vi "Multiprocessing_VI.vi"() -> ()   [LabVIEW 2022 SP3]
uses:
  <vilib>/Analysis/baseanly.llb/Mean (DBL).vi
  <vilib>/DAQmx/read.llb/DAQmx Read (Analog 1D Wfm NChan NSamp).vi
  <vilib>/addons/control/pid/pid.llb/PID Gain Schedule (DBL).vi
  STOP_GLOBAL.vi
  <vilib>/DAQmx/configure/timing.llb/DAQmx Timing (Sample Clock).vi
  <vilib>/DAQmx/miscellaneous.llb/DAQmx Fill In Error Info.vi
  <resource>/objmgr/daqmx.rc
  <vilib>/addons/control/pid/NI_PID_pid.lvlib
  <vilib>/Analysis/NI_AALBase.lvlib
panel:
  in  "Filename":path=path "C:/1. Rocket Research Project/CollectedData/Plots/TestingData.lvm"
  out "Vol Flow":cluster{dbl[], dbl[]}(graph)
  out "Chamber Pressure":cluster{dbl[], dbl[]}(graph)
  out "Inlet Pressure":cluster{dbl[], dbl[]}(graph)
  out "Line Pressure":cluster{dbl[], dbl[]}(graph)
  out "Waveform Chart":cluster{"mean":dbl, "MV":dbl}(graph)
  out "number of samples written per channel":u32
  in  "stop 2":bool
  in  "stop":bool
  out "Voltage Out Array":dbl[](array[numeric])
  out "SampClk.Rate 2":dbl
  out "Output":dbl(slide)=30.8641975308642 scale=0.0..5.067 scale format="%.1f"
  in  "Automatic":bool=TRUE
  in  "SP":dbl
  in  "MV":dbl(slide)=30.8641975308642 scale=0.0..5.067 scale format="%.1f"
  in  "PID gain schedule":T1(array[cluster])=[{"PID gains"={"proportional gain (Kc)"=1.0, "integral time (Ti, min)"=0.01, "derivative time (Td, min)"=0.0}, "max value"=100.0}] {"max value" format="%.2f"; "PID gains"."derivative time (Td, min)" format="%.3f"; "PID gains"."integral time (Ti, min)" format="%.3f"; "PID gains"."proportional gain (Kc)" format="%.3f"}
  out "Supply Pressure":dynamicdata(graph)
  out "Inlet Pressure":dynamicdata(graph)
  out "Line Pressure":dynamicdata(graph)
  out "Chamber Pressure PSI":dynamicdata(graph)
  out "Waiting \nfor Start":bool=TRUE
  in  "Start VI":bool
  out "SampClk.Rate":dbl
  in  "Sample Number":i32=100
  in  "Channel Control":bool[](array[boolean])
  in  "Rate":dbl=1000.0 format="%0.2f"
  out "Time":dbl
  out "Supply Pressure":cluster{dbl[], dbl[]}(graph)
  out "x*y":i32
  out "error out":errorcluster
  out "Iterations":i32
  in  "Collect?":bool=TRUE caption="Enable"
  out "Thrust 3":dynamicdata(graph)
  out "Thrust 2":dynamicdata(graph)
  out "Vertical Stand Thrust":dynamicdata(graph)
  out "AI7":dynamicdata(graph)
  out "AI6":dynamicdata(graph)
  out "AI5":dynamicdata(graph)
  out "Voltage Output":dynamicdata(graph)
  out "Temperature":dynamicdata(graph)
  out "Vol Flow L/min":dynamicdata(graph)
  in  "main":bool
  # "Pressure Channels"
  # "DAQ Configuration"
  # "AI 0 - Supply Pressure"
  # "AI 1 - Line Pressure"
  # "AI 2 - Inlet Pressure"
  # "AI 3 - Chamber Pressure"
  # "AI 4 - Volumetric Flow"
  # "AI 5"
  # "AI 6"
  # "AI 7 - Voltage"
  # "Thrust 1"
  # "Thrust 2"
  # "Thrust 3"
  # "Temperature"
  # "Thrust Channels"
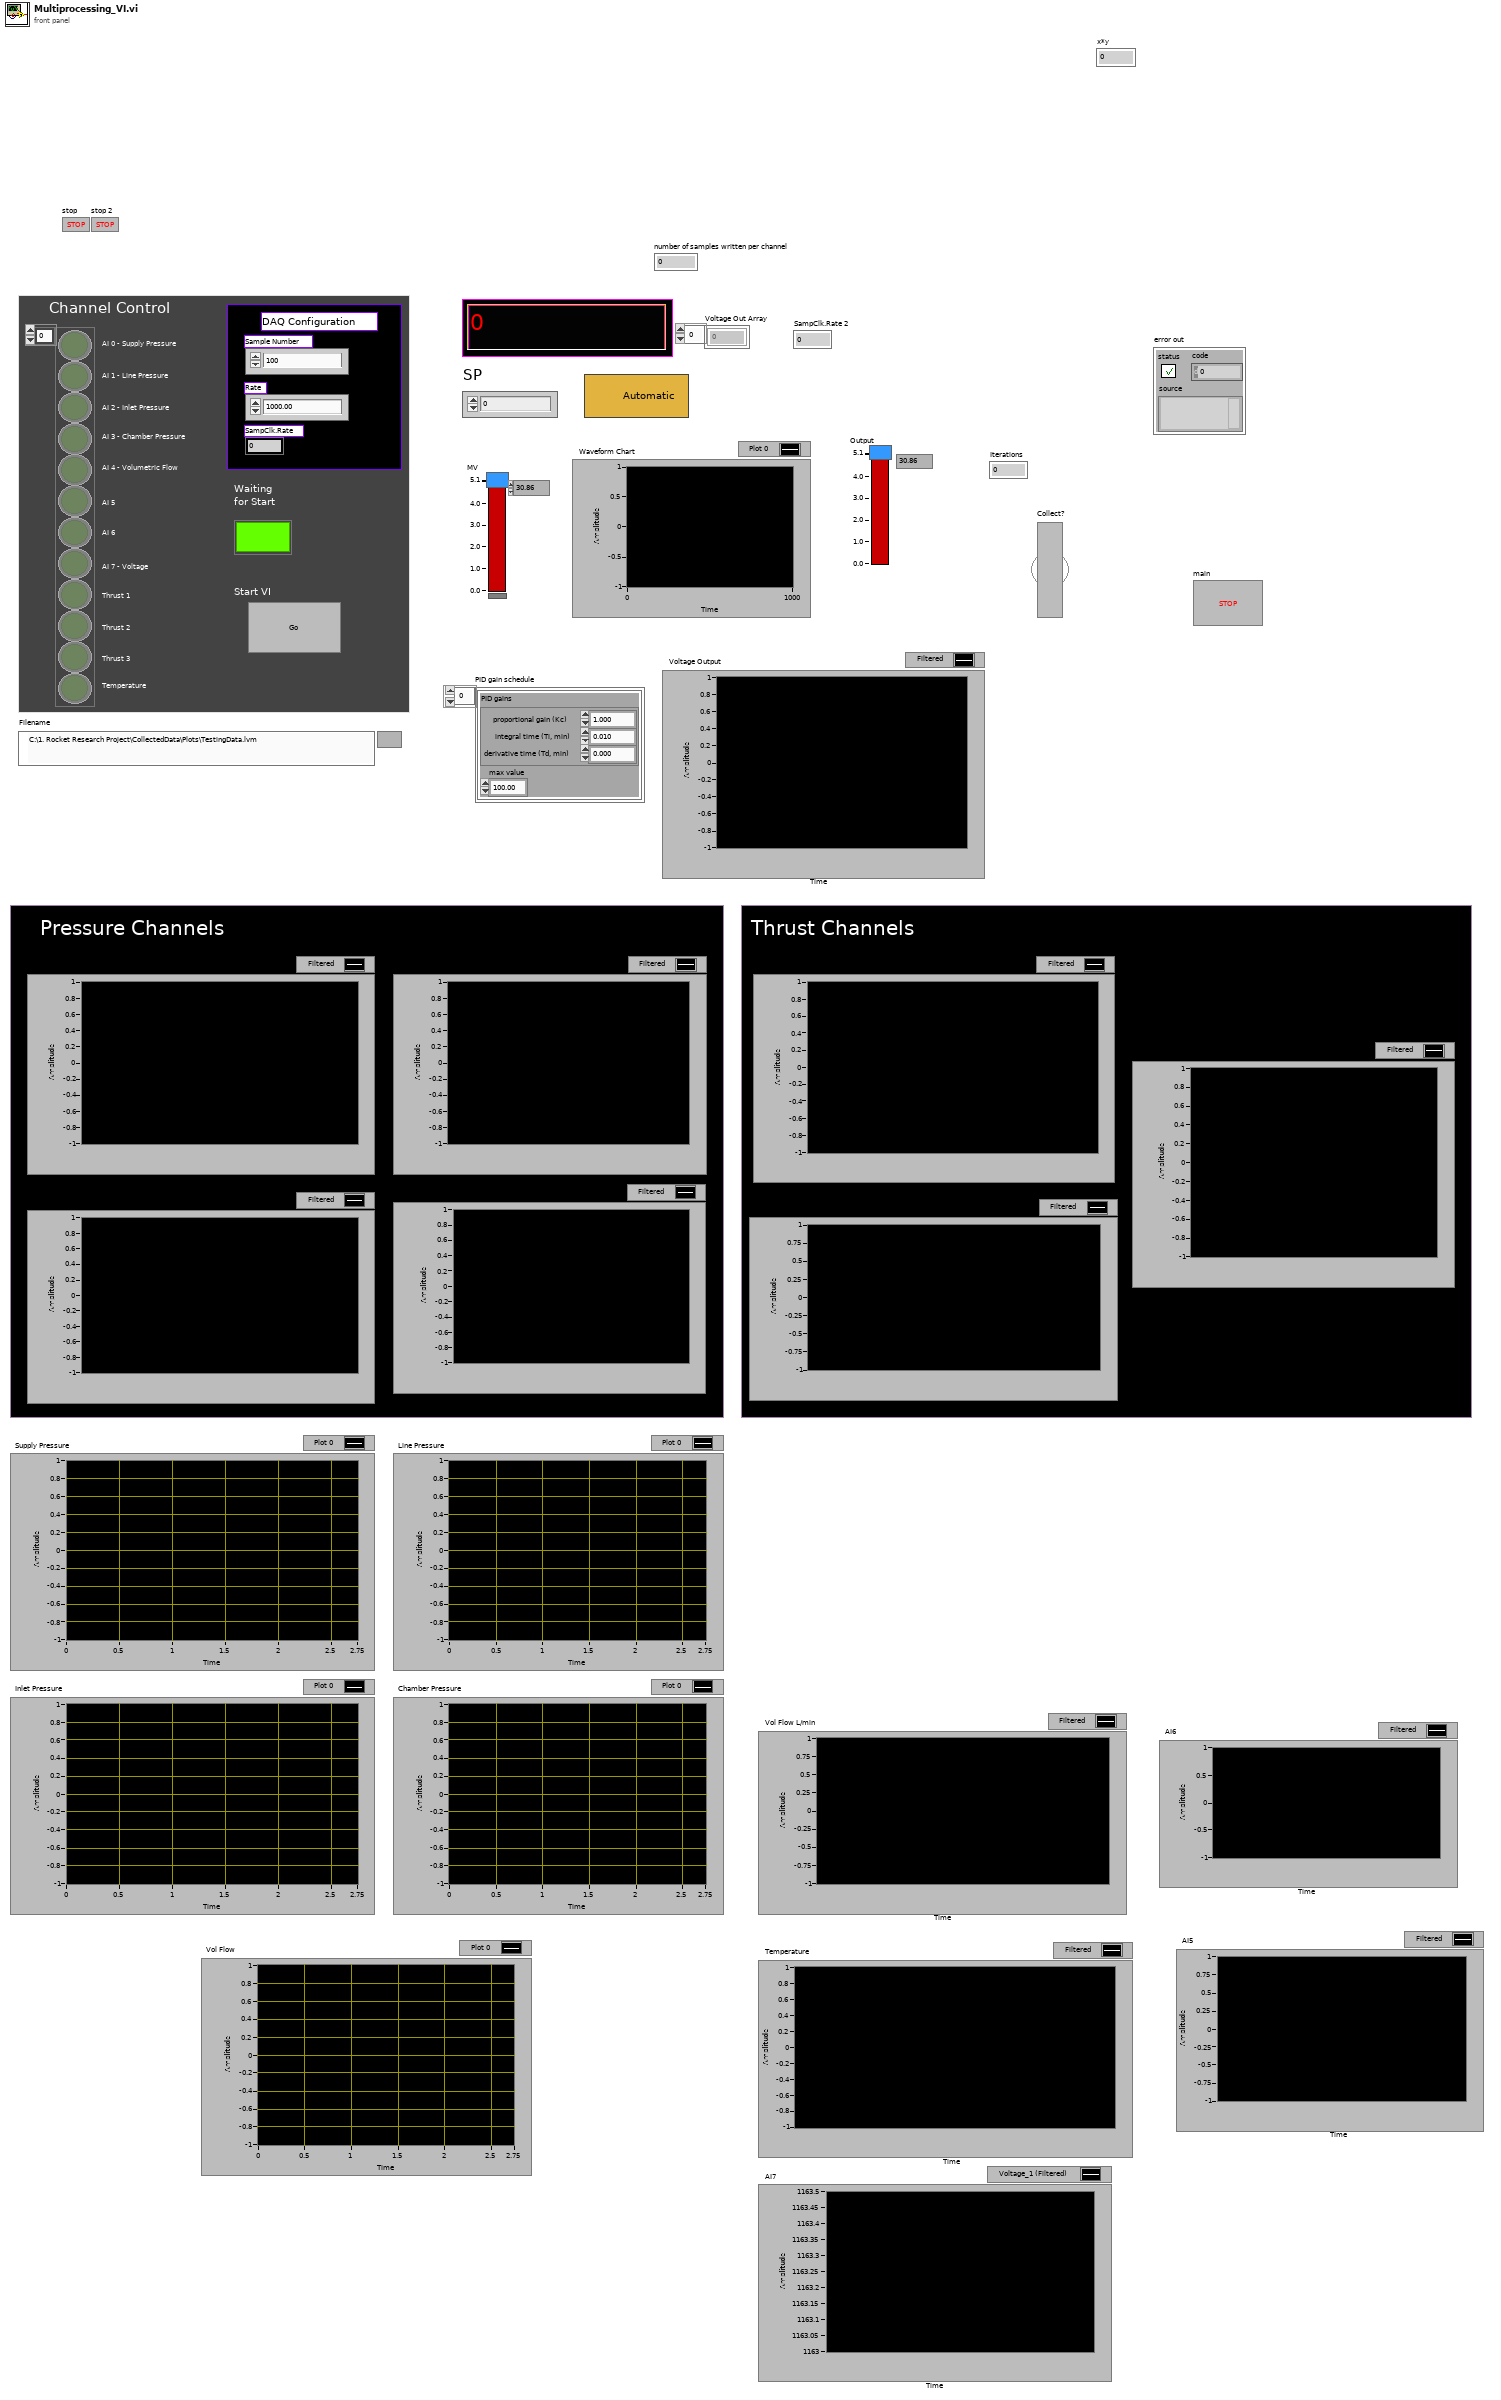
[diagram p1: front panel]
types:
  T1 = cluster{"PID gains":cluster{"proportional gain (Kc)":dbl, "integral time (Ti, min)":dbl, "derivative time (Td, min)":dbl}, "max value":dbl}[]
  T2 = cluster{"Modulus":dbl, "Number of\nComplete Cycles":dbl}
  T3 = cluster{"Dynamic Data":dynamicdata, "Dynamic Data":dynamicdata, "Dynamic Data":dynamicdata, "Dynamic Data":dynamicdata, "Dynamic Data":dynamicdata, "Dynamic Data":dynamicdata, "Dynamic Data":dynamicdata, "Dynamic Data":dynamicdata, "Dynamic Data":dynamicdata, "Dynamic Data":dynamicdata, "Dynamic Data":dynamicdata, "Dynamic Data":dynamicdata}
  T4 = cluster{"PID gains":cluster{"Kc":dbl, "Ti":dbl, "Td":dbl}, "max value":dbl}[]
  T5 = cluster{"proportional gain (Kc)":dbl, "integral time (Ti, min)":dbl, "derivative time (Td, min)":dbl}
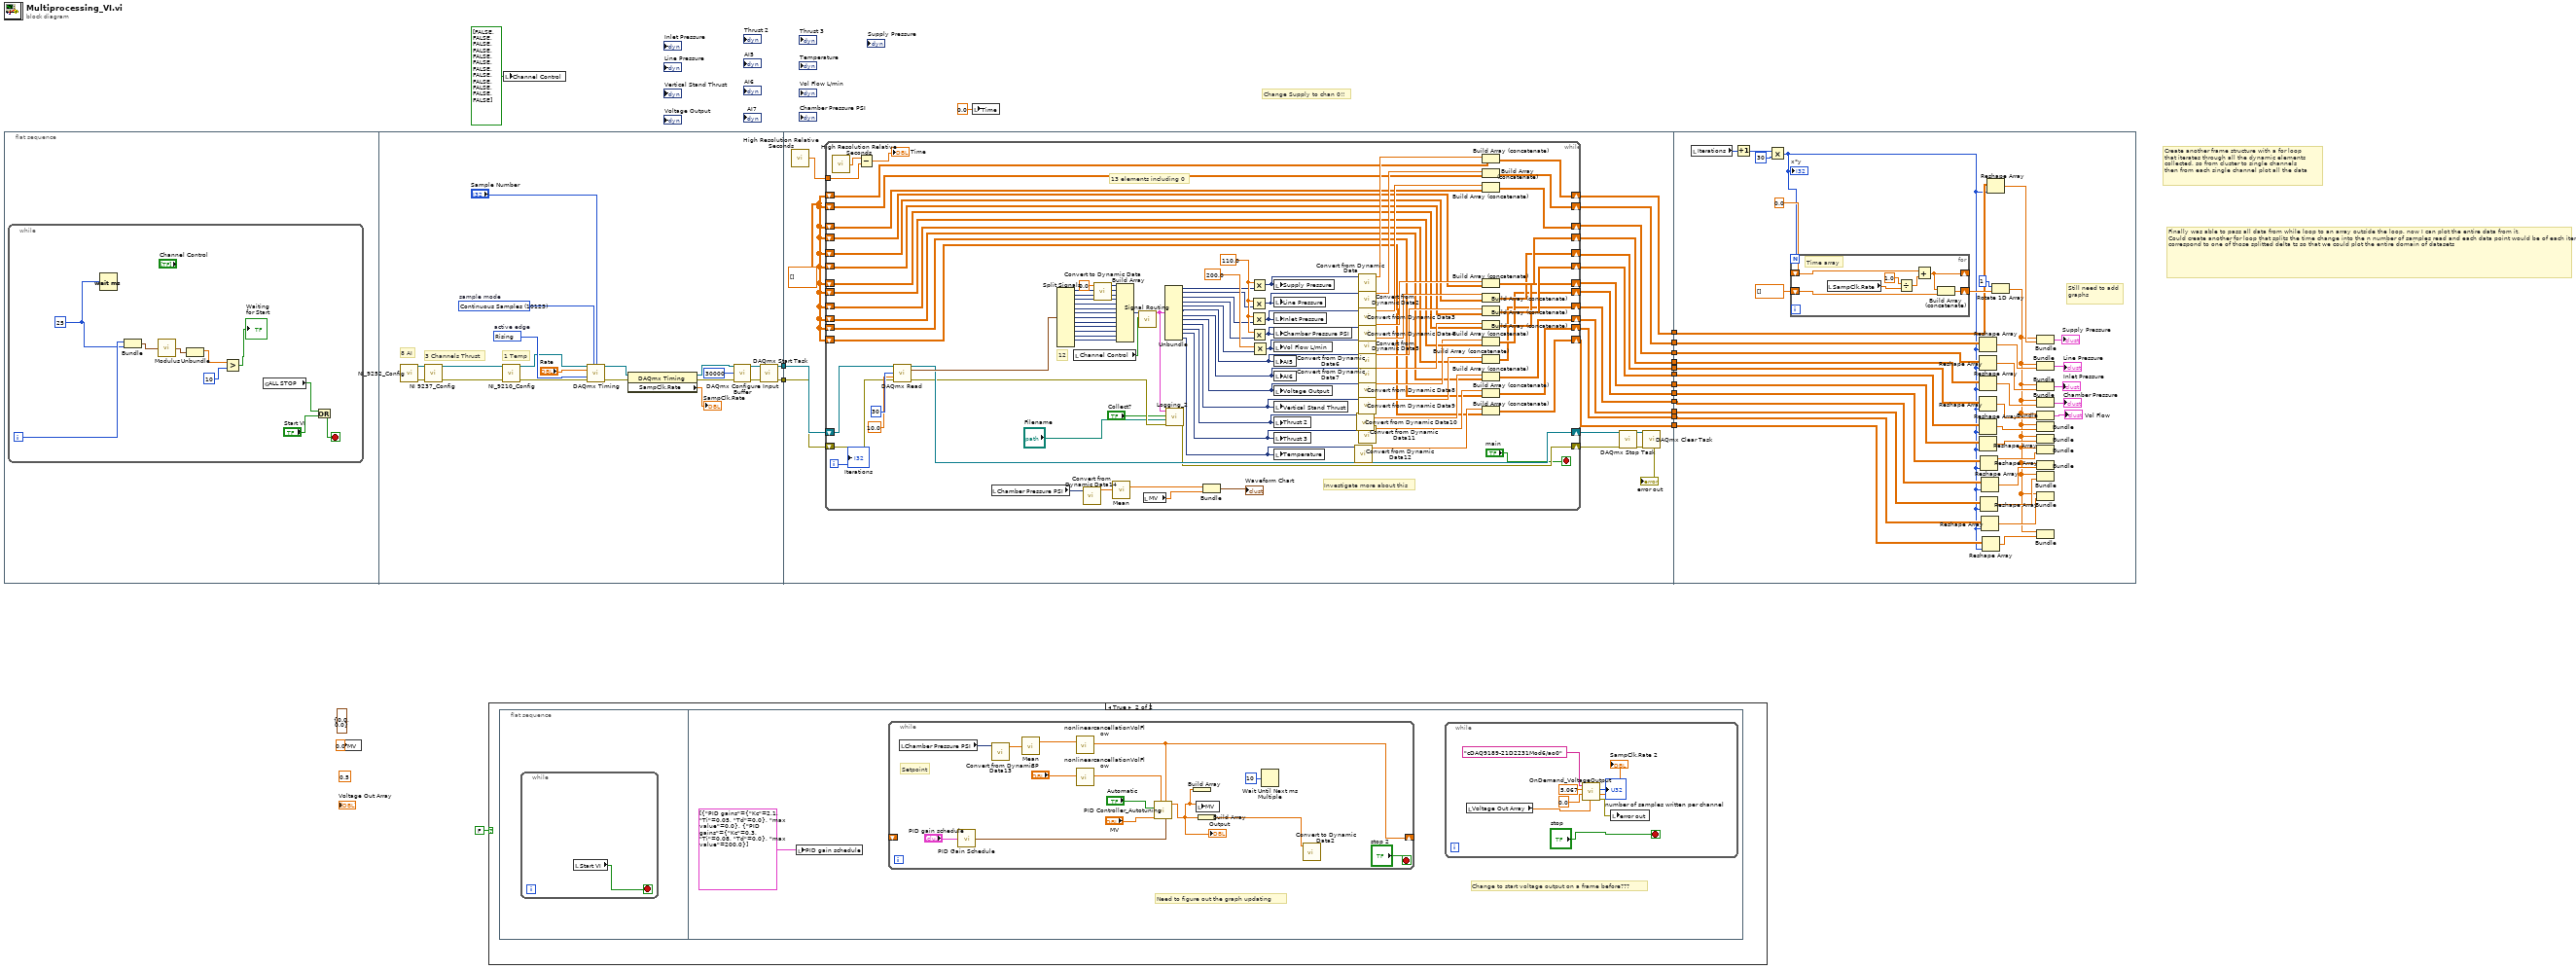
[diagram p0: block diagram]
diagram:
  (unwired) cluster{"initial PV":dbl, "setpoint":dbl} {"initial PV"=0.0, "setpoint"=0.0} ("PV Setpoint Output")
  (unwired) 0.5 ("X Scale.Offset and Multiplier:Multiplier")
  # "Change Supply to chan 0!!"
  # "Finally was able to pass all data from while loop to an array outside the loop, now I can plot the entire data from it, \nCould create another for loop that splits the time change into the n number of samples read and each data point would be of each iteration would correspond to one of those splitted delta ts so that we could plot the entire domain of datasets"
  # "Create another frame structure with a for loop\nthat iterates through all the dynamic elements\ncollected, so from cluster to single channels\nthen from each single channel plot all the data"
  n1 = flat-sequence {
    tunnel: [w34] -> w17
    tunnel: [w33] -> w16
    tunnel: w17 -> [w69]
    tunnel: w16 -> [w68]
    tunnel: [w61] -> w15
    tunnel: [w59] -> w13
    tunnel: [w58] -> w12
    tunnel: [w57] -> w11
    tunnel: [w56] -> w10
    tunnel: [w55] -> w9
    tunnel: [w54] -> w8
    tunnel: [w53] -> w7
    tunnel: [w52] -> w6
    tunnel: [w51] -> w5
    tunnel: [w50] -> w4
    tunnel: [w49] -> w3
    tunnel: w15 -> [w190]
    tunnel: w13 -> [w189]
    tunnel: w12 -> [w188]
    tunnel: w11 -> [w187]
    tunnel: w10 -> [w186]
    tunnel: w9 -> [w185]
    tunnel: w8 -> [w184]
    tunnel: w7 -> [w177]
    tunnel: w6 -> [w175]
    tunnel: w5 -> [w173]
    tunnel: w4 -> [w171]
    tunnel: w3 -> [w167]
    frame #0 {
      n2 = while {
        i -> [w28]
        stop <- w20 stop-if-true
        w19 = u32 25 ("milliseconds to wait")
        n3 = Wait (ms)(milliseconds to wait=w19) -> ()  [unwired: 1 out]
        n4 = Bundle(w28, "milliseconds to wait"=w19) -> (w27:cluster{i32, "milliseconds to wait":u32})  [unwired: 1 in]
        n5 = call "Modulus.vi"("Input"=w27) -> ("Output"=w26:T2)
        n6 = Unbundle(w26) -> ("Modulus"=w25:dbl)  [unwired: 1 out]
        n7 = Greater?(x=w25, y=u32 10 ("milliseconds to wait")) -> (0:→"Waiting \nfor Start":bool)
        n8 = global read "STOP_GLOBAL.vi" "ALL STOP"() -> (w22:bool)
        n9 = Or(x=w22, y="Start VI") -> (x .or. y?=w20:bool)
      }
    }
    frame #1 {
      w38 = 10123 items=["Finite Samples"=10178, "Continuous Samples"=10123, "Hardware Timed Single Point"=12522]  # sample mode
      w37 = 10280 items=["Rising"=10280, "Falling"=10171]  # active edge
      # "1 Temp"
      # "8 AI"
      # "3 Channels Thrust"
      n10 = call "NI_9252_Config.vi"() -> ("error out"=w31:errorcluster, "task out"=w32:refnum<k21>)  [unwired: 10 in]
      n11 = call "NI 9237_Config.vi"("error in"=w31, "task in"=w32) -> ("error out"=w48:errorcluster, "task out"=w47:refnum<k21>)  [unwired: 8 in]
      n12 = call "NI_9210_Config.vi"("error in"=w48, "task in"=w47) -> ("error out"=w30:errorcluster, "task out"=w29:refnum<k21>)  [unwired: 8 in]
      n13 = call-poly <vilib>:"DAQmx Timing.vi"("task/channels in"=w29, "sample mode"=w38, "samples per channel"="Sample Number", "rate"="Rate", "active edge"=w37, "error in"=w30) -> ("task out"=w41:refnum<k21>, "error out"=w42:errorcluster)  [unwired: 8 in]
      n14 = property class="DAQmx Timing"(reference=w41, error in=w42) -> (reference out=w43:refnum<k21>, error out=w44:errorcluster, "SampClk.Rate"=→"SampClk.Rate":dbl)
      n15 = call <vilib>:"DAQmx Configure Input Buffer.vi"("task/channels in"=w43, "buffer size (in samples per channel)"=u32 30000, "error in"=w44) -> ("task out"=w46:refnum<k21>, "error out"=w45:errorcluster)  [unwired: 11 in]
      n16 = call <vilib>:"DAQmx Start Task.vi"("task/channels in"=w46, "error in"=w45) -> ("task out"=w34:refnum<k21>, "error out"=w33:errorcluster)  [unwired: 12 in]
    }
    frame #2 {
      w60 = dbl[][] []
      n17 = call <vilib>:"High Resolution Relative Seconds.vi"() -> ("relative seconds"=w67:dbl)
      n18 = while {
        shift-right: [w156] -> w63
        shift-left: w69 -> [w158]
        shift-right: [w131] -> w62
        shift-left: w68 -> [w157]
        shift-right: [w123] -> w61
        shift-left: w60 -> [w76]
        tunnel: w67 -> [w126]
        shift-right: [w117] -> w59
        shift-left: w60 -> [w118]
        shift-right: [w111] -> w58
        shift-left: w60 -> [w112]
        shift-right: [w109] -> w57
        shift-left: w60 -> [w110]
        shift-right: [w106] -> w56
        shift-left: w60 -> [w105]
        shift-right: [w99] -> w55
        shift-left: w60 -> [w97]
        shift-right: [w98] -> w54
        shift-left: w60 -> [w96]
        shift-right: [w95] -> w53
        shift-left: w60 -> [w94]
        shift-right: [w88] -> w52
        shift-left: w60 -> [w87]
        shift-right: [w86] -> w51
        shift-left: w60 -> [w85]
        shift-right: [w82] -> w50
        shift-left: w60 -> [w81]
        shift-right: [w78] -> w49
        shift-left: w60 -> [w77]
        i -> [w129]
        stop <- "main" stop-if-true
        w139 = 110.0 ("x")
        # "Investigate more about this"
        # "13 elements including 0"
        # "12"
        n19 = call <vilib>:"High Resolution Relative Seconds.vi"() -> ("relative seconds"=w127:dbl)
        n20 = Subtract(x=w127, y=w126) -> (x-y=→"Time":dbl)
        n21 = call-poly <vilib>:"DAQmx Read.vi"("task/channels in"=w158, "number of samples per channel"=30, "timeout"=10.0, "error in"=w157) -> ("task out"=w156:refnum<k21>, "data"=w159:waveform(dbl)[], "error out"=w133:errorcluster)  [unwired: 9 in]
        n22 = local read "Chamber Pressure PSI"() -> (w74:dynamicdata)
        n23 = Split Signals(w159) -> (w150:dynamicdata, w155:dynamicdata, w154:dynamicdata, w153:dynamicdata, w152:dynamicdata, w151:dynamicdata, w149:dynamicdata, w148:dynamicdata, w147:dynamicdata, w146:dynamicdata, w145:dynamicdata, w142:dynamicdata)  [unwired: 13 in, 1 out]
        n24 = local read "Channel Control"() -> (w141:bool[])
        n25 = call "Convert from Dynamic Data14"("Dynamic Data Type"=w74) -> ("Array"=w75:dbl[])  [unwired: 3 in]
        n26 = call "Convert to Dynamic Data"("Double"=0.0) -> ("Dynamic Data Type"=w143:dynamicdata)  [unwired: 3 in]
        n27 = call-poly <vilib>:"Mean.vi"("X"=w75) -> ("mean"=w73:dbl)  [unwired: 1 out]
        n28 = Build Array(w143, w150, w155, w154, w153, w152, w151, w149, w148, w147, w146, w145, w142) -> (w140:dynamicdata[])
        n29 = call "Signal Routing.vi"("Boolean Array"=w141, "Data In"=w140) -> ("Output"=w128:T3)  [unwired: 9 in]
        n30 = local read "MV"() -> (w72:dbl)
        n31 = Unbundle(w128) -> ("Dynamic Data"=w130:dynamicdata, "Dynamic Data"=w137:dynamicdata, "Dynamic Data"=w136:dynamicdata, "Dynamic Data"=w135:dynamicdata, "Dynamic Data"=w134:dynamicdata, "Dynamic Data"=w104:dynamicdata, "Dynamic Data"=w103:dynamicdata, "Dynamic Data"=w102:dynamicdata, "Dynamic Data"=w93:dynamicdata, "Dynamic Data"=w89:dynamicdata, "Dynamic Data"=w84:dynamicdata, "Dynamic Data"=w79:dynamicdata)
        n32 = call "Logging_2.vi"("error in"=w133, "Filename"="Filename", "Enable"="Collect?", "output cluster"=w128) -> ("error out"=w131:errorcluster)  [unwired: 7 in]
        n33 = Bundle("mean"=w73, "MV"=w72) -> (→"Waveform Chart":cluster{"mean":dbl, "MV":dbl})  [unwired: 1 in]
        n34 = Multiply(x=w139, y=w137) -> (x*y=w120:dynamicdata)
        n35 = Multiply(x=w139, y=w136) -> (x*y=w116:dynamicdata)
        n36 = Multiply(x=w139, y=w130) -> (x*y=w125:dynamicdata)
        n37 = Multiply(x=w139, y=w135) -> (x*y=w115:dynamicdata)
        n38 = Multiply(x=200.0, y=w134) -> (x*y=w108:dynamicdata)
        n39 = local write "Supply Pressure"(w125) -> ()
        n40 = local write "Line Pressure"(w120) -> ()
        n41 = local write "Inlet Pressure"(w116) -> ()
        n42 = local write "Chamber Pressure PSI"(w115) -> ()
        n43 = local write "Vol Flow L/min"(w108) -> ()
        n44 = local write "AI5"(w104) -> ()
        n45 = local write "AI6"(w103) -> ()
        n46 = local write "Voltage Output"(w102) -> ()
        n47 = local write "Vertical Stand Thrust"(w93) -> ()
        n48 = local write "Thrust 2"(w89) -> ()
        n49 = local write "Thrust 3"(w84) -> ()
        n50 = local write "Temperature"(w79) -> ()
        n51 = call "Convert from Dynamic Data12"("Dynamic Data Type"=w79) -> ("Array"=w80:dbl[])  [unwired: 3 in]
        n52 = call "Convert from Dynamic Data10"("Dynamic Data Type"=w89) -> ("Array"=w90:dbl[])  [unwired: 3 in]
        n53 = call "Convert from Dynamic Data"("Dynamic Data Type"=w125) -> ("Array"=w124:dbl[])  [unwired: 3 in]
        n54 = call "Convert from Dynamic Data2"("Dynamic Data Type"=w120) -> ("Array"=w119:dbl[])  [unwired: 3 in]
        n55 = call "Convert from Dynamic Data3"("Dynamic Data Type"=w116) -> ("Array"=w114:dbl[])  [unwired: 3 in]
        n56 = call "Convert from Dynamic Data4"("Dynamic Data Type"=w115) -> ("Array"=w113:dbl[])  [unwired: 3 in]
        n57 = call "Convert from Dynamic Data5"("Dynamic Data Type"=w108) -> ("Array"=w107:dbl[])  [unwired: 3 in]
        n58 = call "Convert from Dynamic Data6"("Dynamic Data Type"=w104) -> ("Array"=w101:dbl[])  [unwired: 3 in]
        n59 = call "Convert from Dynamic Data7"("Dynamic Data Type"=w103) -> ("Array"=w100:dbl[])  [unwired: 3 in]
        n60 = call "Convert from Dynamic Data8"("Dynamic Data Type"=w102) -> ("Array"=w92:dbl[])  [unwired: 3 in]
        n61 = call "Convert from Dynamic Data9"("Dynamic Data Type"=w93) -> ("Array"=w91:dbl[])  [unwired: 3 in]
        n62 = call "Convert from Dynamic Data11"("Dynamic Data Type"=w84) -> ("Array"=w83:dbl[])  [unwired: 3 in]
        n63 = Build Array (concatenate)(w124, w76) -> (w123:dbl[][])
        n64 = Build Array (concatenate)(w119, w118) -> (w117:dbl[][])
        n65 = Build Array (concatenate)(w114, w112) -> (w111:dbl[][])
        n66 = Build Array (concatenate)(w113, w110) -> (w109:dbl[][])
        n67 = Build Array (concatenate)(w107, w105) -> (w106:dbl[][])
        n68 = Build Array (concatenate)(w101, w97) -> (w99:dbl[][])
        n69 = Build Array (concatenate)(w100, w96) -> (w98:dbl[][])
        n70 = Build Array (concatenate)(w92, w94) -> (w95:dbl[][])
        n71 = Build Array (concatenate)(w91, w87) -> (w88:dbl[][])
        n72 = Build Array (concatenate)(w90, w85) -> (w86:dbl[][])
        n73 = Build Array (concatenate)(w83, w81) -> (w82:dbl[][])
        n74 = Build Array (concatenate)(w80, w77) -> (w78:dbl[][])
        "Iterations" <- w129
      }
      n75 = call <vilib>:"DAQmx Stop Task.vi"("task/channels in"=w63, "error in"=w62) -> ("task out"=w66:refnum<k21>, "error out"=w65:errorcluster)  [unwired: 12 in]
      n76 = call <vilib>:"DAQmx Clear Task.vi"("task in"=w66, "error in"=w65) -> ("error out"=→"error out":errorcluster)  [unwired: 13 in]
    }
    frame #3 {
      # "Still need to add\ngraphs"
      n77 = local read "Iterations"() -> (w198:i32)
      n78 = Increment(x=w198) -> (x+1=w197:i32)
      n79 = Multiply(x=w197, y=30 ("number of samples per channel")) -> (x*y=w166:i32)
      "x*y" <- w166
      n80 = for {
        N: w166 -> [_]
        shift-right: [w202] -> _
        shift-left: 0.0 -> [w203]
        shift-right: [w201] -> w194
        shift-left: dbl[] [] -> [w200]
        # "Time array"
        n81 = local read "SampClk.Rate"() -> (w205:dbl)
        n82 = Divide(x=1.0, y=w205) -> (x/y=w204:dbl)
        n83 = Add(x=w203, y=w204) -> (x+y=w202:dbl)
        n84 = Build Array (concatenate)(w202, w200) -> (w201:dbl[])
      }
      n85 = Reshape Array(w189, w166) -> (w183:dbl[])
      n86 = Reshape Array(w188, w166) -> (w182:dbl[])
      n87 = Reshape Array(w187, w166) -> (w181:dbl[])
      n88 = Reshape Array(w186, w166) -> (w180:dbl[])
      n89 = Reshape Array(w185, w166) -> (w179:dbl[])
      n90 = Reshape Array(w184, w166) -> (w178:dbl[])
      n91 = Reshape Array(w177, w166) -> (w176:dbl[])
      n92 = Reshape Array(w173, w166) -> (w172:dbl[])
      n93 = Reshape Array(w175, w166) -> (w174:dbl[])
      n94 = Reshape Array(w171, w166) -> (w170:dbl[])
      n95 = Reshape Array(w167, w166) -> (w168:dbl[])
      n96 = Reshape Array(w190, w166) -> (w192:dbl[])
      n97 = Rotate 1D Array(1:w194, 2:1 ("n")) -> (0:w169:dbl[])
      n98 = Bundle(w169, w192) -> (→"Supply Pressure":cluster{dbl[], dbl[]})  [unwired: 1 in]
      n99 = Bundle(w169, w183) -> (→"Line Pressure":cluster{dbl[], dbl[]})  [unwired: 1 in]
      n100 = Bundle(w169, w182) -> (→"Inlet Pressure":cluster{dbl[], dbl[]})  [unwired: 1 in]
      n101 = Bundle(w169, w181) -> (→"Chamber Pressure":cluster{dbl[], dbl[]})  [unwired: 1 in]
      n102 = Bundle(w169, w180) -> (→"Vol Flow":cluster{dbl[], dbl[]})  [unwired: 1 in]
      n103 = Bundle(w169, w179) -> ()  [unwired: 1 in, 1 out]
      n104 = Bundle(w169, w178) -> ()  [unwired: 1 in, 1 out]
      n105 = Bundle(w169, w176) -> ()  [unwired: 1 in, 1 out]
      n106 = Bundle(w169, w174) -> ()  [unwired: 1 in, 1 out]
      n107 = Bundle(w169, w172) -> ()  [unwired: 1 in, 1 out]
      n108 = Bundle(w169, w170) -> ()  [unwired: 1 in, 1 out]
      n109 = Bundle(w169, w168) -> ()  [unwired: 1 in, 1 out]
    }
  }
  n110 = local write "MV"(0.0 ("MV")) -> ()
  n111 = case shown="True" FALSE {
    frame False {
    }
    frame True {
      n112 = flat-sequence {
        frame #0 {
          n113 = while {
            stop <- w207 stop-if-true
            n114 = local read "Start VI"() -> (w207:bool)
          }
        }
        frame #1 {
          # "Need to figure out the graph updating"
          # "Change to start voltage output on a frame before???"
          n115 = local write "PID gain schedule"(T4 [{"PID gains"={"Kc"=2.1, "Ti"=0.05, "Td"=0.0}, "max value"=0.0}, {"PID gains"={"Kc"=0.3, "Ti"=0.08, "Td"=0.0}, "max value"=200.0}]) -> ()
          n116 = while {
            shift-right: [w226] -> _
            shift-left: _ -> [_]
            stop <- "stop 2" stop-if-true
            # "Setpoint"
            n117 = local read "Chamber Pressure PSI"() -> (w218:dynamicdata)
            n118 = call-poly <vilib>:"PID Gain Schedule.vi"("PID gain schedule"="PID gain schedule") -> ("PID gains out"=w227:T5)  [unwired: 3 in, 1 out]
            n119 = call "Convert from Dynamic Data13"("Dynamic Data Type"=w218) -> ("Array"=w230:dbl[])  [unwired: 3 in]
            n120 = call-poly <vilib>:"Mean.vi"("X"=w230) -> ("mean"=w229:dbl)  [unwired: 1 out]
            n121 = call "nonlinearcancellationVolFlow.vi"("input variable"=w229) -> ("MVT Process Variable"=w226:dbl)  [unwired: 10 in]
            n122 = call "nonlinearcancellationVolFlow.vi"("input variable"="SP") -> ("MVT Process Variable"=w224:dbl)  [unwired: 10 in]
            n123 = call "PID Controller_Autotuning.vi"("PID gains in"=w227, "process variable"=w226, "setpoint"=w224, "manipulated variable"="MV", "Automatic"="Automatic") -> ("output"=w219:dbl)  [unwired: 5 in, 1 out]
            "Output" <- w219
            n124 = Build Array(w219) -> ()  [unwired: 1 out]
            n125 = local write "MV"(w219) -> ()
            n126 = Build Array(w219) -> (w221:dbl[])
            n127 = Wait Until Next ms Multiple(millisecond multiple=u32 10) -> ()  [unwired: 1 out]
            n128 = call "Convert to Dynamic Data2"("Array"=w221) -> ()  [unwired: 3 in, 1 out]
          }
          n129 = while {
            stop <- "stop" stop-if-true
            n130 = local read "Voltage Out Array"() -> (w211:dbl[])
            n131 = call "OnDemand_VoltageOutput.vi"("Channel Array"=w211, "minimum voltage"=0.0, "maximum voltage"=5.067, "physical channels"="cDAQ9189-21D2231Mod6/ao0") -> ("error out"=w212:errorcluster, "SampClk.Rate"=→"SampClk.Rate 2":dbl, "number of samples written per channel"=→"number of samples written per channel":u32)  [unwired: 5 in]
            n132 = local write "error out"(w212) -> ()
          }
        }
      }
    }
  }
  n133 = local write "Channel Control"(bool[] [FALSE, FALSE, FALSE, FALSE, FALSE, FALSE, FALSE, FALSE, FALSE, FALSE, FALSE, FALSE] ("Array")) -> ()
  n134 = local write "Time"(0.0 ("Time")) -> ()
